vi "Clear.vi"(8 "error in (no error)":errorcluster caption="错误输入（无错误）", 11 "Dictionary In":refnum<class "Dictionary.lvclass"> caption="DNL_LabVIEW Object in") -> (0 "error out":errorcluster caption="错误输出", 3 "Dictionary Out":refnum<class "Dictionary.lvclass"> caption="DNL_LabVIEW Object out")   [LabVIEW 2012, in "Dictionary.lvclass"]
uses:
  Dictionary.lvclass
  Dictionary.lvclass/Dictionary.ctl
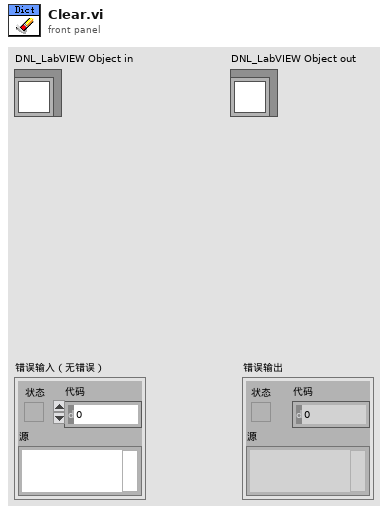
[diagram p1: front panel]
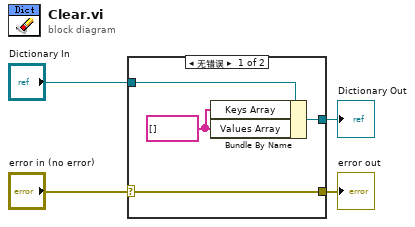
[diagram p0: block diagram]
diagram:
  n1 = case shown="无错误" "error in (no error)" {
    selector: "error in (no error)" -> [w8 w10]
    tunnel: [w8 w10] -> w3
    tunnel: [w6 w9] -> w1
    tunnel: "Dictionary In" -> [w7 w9]
    frame No Error {
      w5 = string[] [] ("Keys Array")
      n2 = Bundle By Name(cluster=w7, "Keys Array"=w5, "Values Array"=w5) -> (w6:refnum<class "Dictionary.lvclass">)
    }
    frame Error {
    }
  }
  "error out" <- w3
  "Dictionary Out" <- w1
